vi "DDM Process Digital Data.vi"(0 "Captured Digital Waveform In":digitalwaveform[](array[waveform]), 11 "error in (no error)":errorcluster) -> (4 "Digital Waveform Out":digitalwaveform(waveform), 6 "Port Digital Data":u32[](array[numeric]), 15 "error out":errorcluster)   [LabVIEW 2021, in "DAQ_Dynamic Digital Pattern Measurement.lvlib"]
doc: "Processes the captured 1D Digital waveform data where digital lines are presented in each array elements into a single Digital waveform format where all digital lines data are appended in consecutive MSB bits."
uses:
  DAQ_Dynamic Digital Pattern Measurement.lvlib
  <vilib>/Waveform/DWDTOps.llb/DWDT Append Digital Signals.vi
  <vilib>/Waveform/DWDTOps.llb/DWDT Digital to Boolean Array.vi
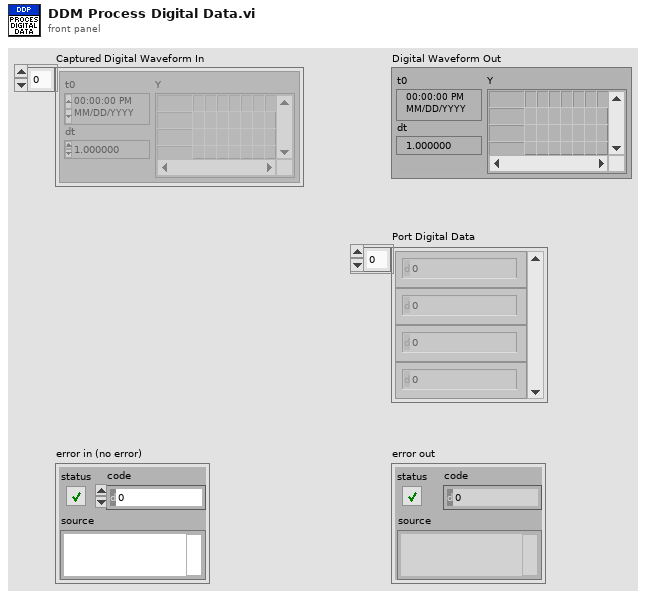
[diagram p1: front panel]
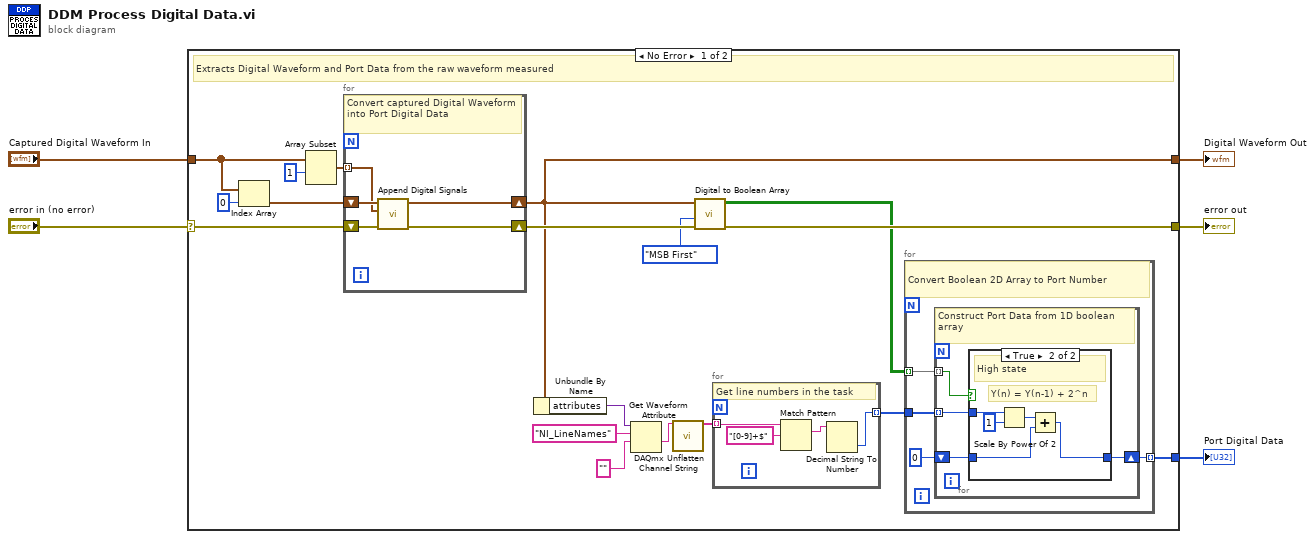
[diagram p0: block diagram]
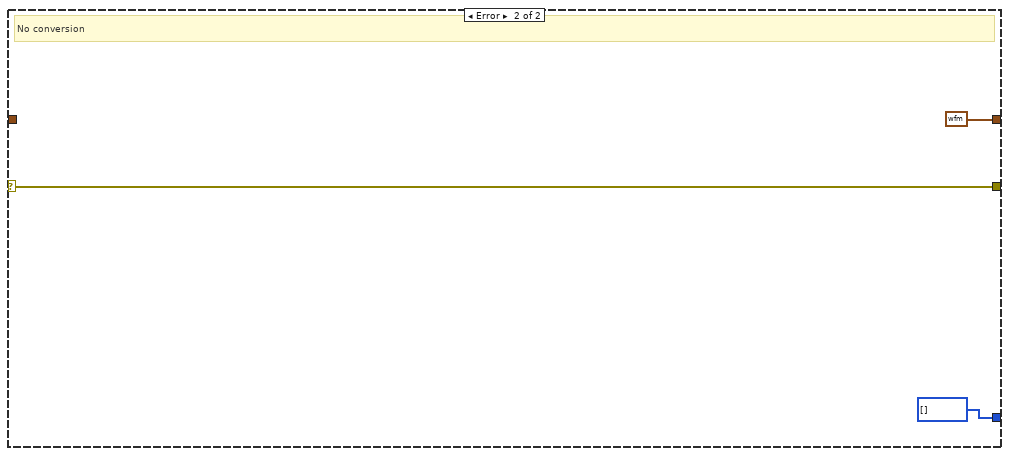
[diagram p3: hidden frame]
diagram:
  n1 = case shown="No Error" "error in (no error)" {
    selector: "error in (no error)" -> [w23 w49]
    tunnel: "Captured Digital Waveform In" -> [w21 _]
    tunnel: [w16 w49] -> w3
    tunnel: [w15 digitalwaveform {"t0"=timestamp(0 s since 1904-01-01), "dt"=0.0, "Y"={"transitions"=[], "data"=[]}} ("Digital Waveform")] -> w2
    tunnel: [w14 u32[] []] -> w1
    frame No Error {
      # "Extracts Digital Waveform and Port Data from the raw waveform measured"
      n2 = Index Array(array=w21, index=0) -> (element=w22:digitalwaveform)
      n3 = Array Subset(array=w21, index=1) -> (w19:digitalwaveform[])  [unwired: 1 in]
      n4 = for {
        shift-right: [w25] -> w17
        shift-left: w23 -> [w28]
        shift-right: [w27] -> w15
        shift-left: w22 -> [w26]
        tunnel: w19 -> [w24] mode=indexing
        # "Convert captured Digital Waveform into Port Digital Data"
        n5 = call-poly <vilib>:"Append Digital Signals.vi"("error in (no error)"=w28, "digital waveform (low bits)"=w24, "digital waveform (high bits)"=w26) -> ("error out"=w25:errorcluster, "digital waveform out"=w27:digitalwaveform)  [unwired: 7 in]
      }
      n6 = Unbundle By Name(w15) -> ("attributes"=w11:variant)
      n7 = Get Waveform Attribute(5:"", 6:"NI_LineNames" ("name"), 7:w11) -> (1:w7:string)  [unwired: 1 in, 3 out]
      n8 = call <vilib>:"DAQmx Unflatten Channel String.vi"("names in"=w7) -> ("names out"=w8:string[])  [unwired: 13 in, 1 out]
      n9 = call-poly <vilib>:"Digital to Boolean Array.vi"("error in (no error)"=w17, "mode"=enum16{"LSB First", "MSB First"}."MSB First", "digital waveform"=w15) -> ("error out"=w16:errorcluster, "boolean array"=w12:bool[][])  [unwired: 7 in]
      n10 = for {
        tunnel: w8 -> [w46] mode=indexing
        tunnel: [w43] -> w6 mode=indexing
        # "Get line numbers in the task"
        n11 = Match Pattern(string=w46, regular expression="[0-9]+$") -> (match substring=w44:string)  [unwired: 1 in, 3 out]
        n12 = Decimal String To Number(string=w44) -> (number=w43:i32)  [unwired: 2 in, 1 out]
      }
      n13 = for {
        tunnel: w12 -> [w32] mode=indexing
        tunnel: w6 -> [w31]
        tunnel: [w29] -> w14 mode=indexing
        # "Convert Boolean 2D Array to Port Number"
        n14 = for {
          tunnel: w32 -> [w33] mode=indexing
          tunnel: w31 -> [w36] mode=indexing
          shift-right: [w34] -> w29
          shift-left: u32 0 -> [w35]
          # "Construct Port Data from 1D boolean array"
          n15 = case shown="True" w33 {
            tunnel: w36 -> [_ w42]
            tunnel: w35 -> [w37 w39]
            tunnel: [w37 w38] -> w34
            frame False {
              # "Low state"
            }
            frame True {
              # "Y(n) = Y(n-1) + 2^n"
              # "High state"
              n16 = Scale By Power Of 2(n=w42, x=u32 1) -> (x*2^n=w40:u32)
              n17 = Add(x=w40, y=w39) -> (x+y=w38:u32)
            }
          }
        }
      }
    }
    frame Error {
      # "No conversion"
    }
  }
  "Digital Waveform Out" <- w2
  "error out" <- w3
  "Port Digital Data" <- w1
